vi "XML Parser Scheds.vi"(8 "error in (no error)":errorcluster, 11 "Schedule Filename":string) -> (0 "error out":errorcluster, 3 "output array":string[][](array[string]))   [LabVIEW 2023]
uses:
  <vilib>/xml/Close Reference(Node).vi
  <vilib>/xml/NI_XML.lvlib
  <resource>/objmgr/DOMUserDefRef.rc
panel:
  out "XML":string
  out "Parse Errors":string
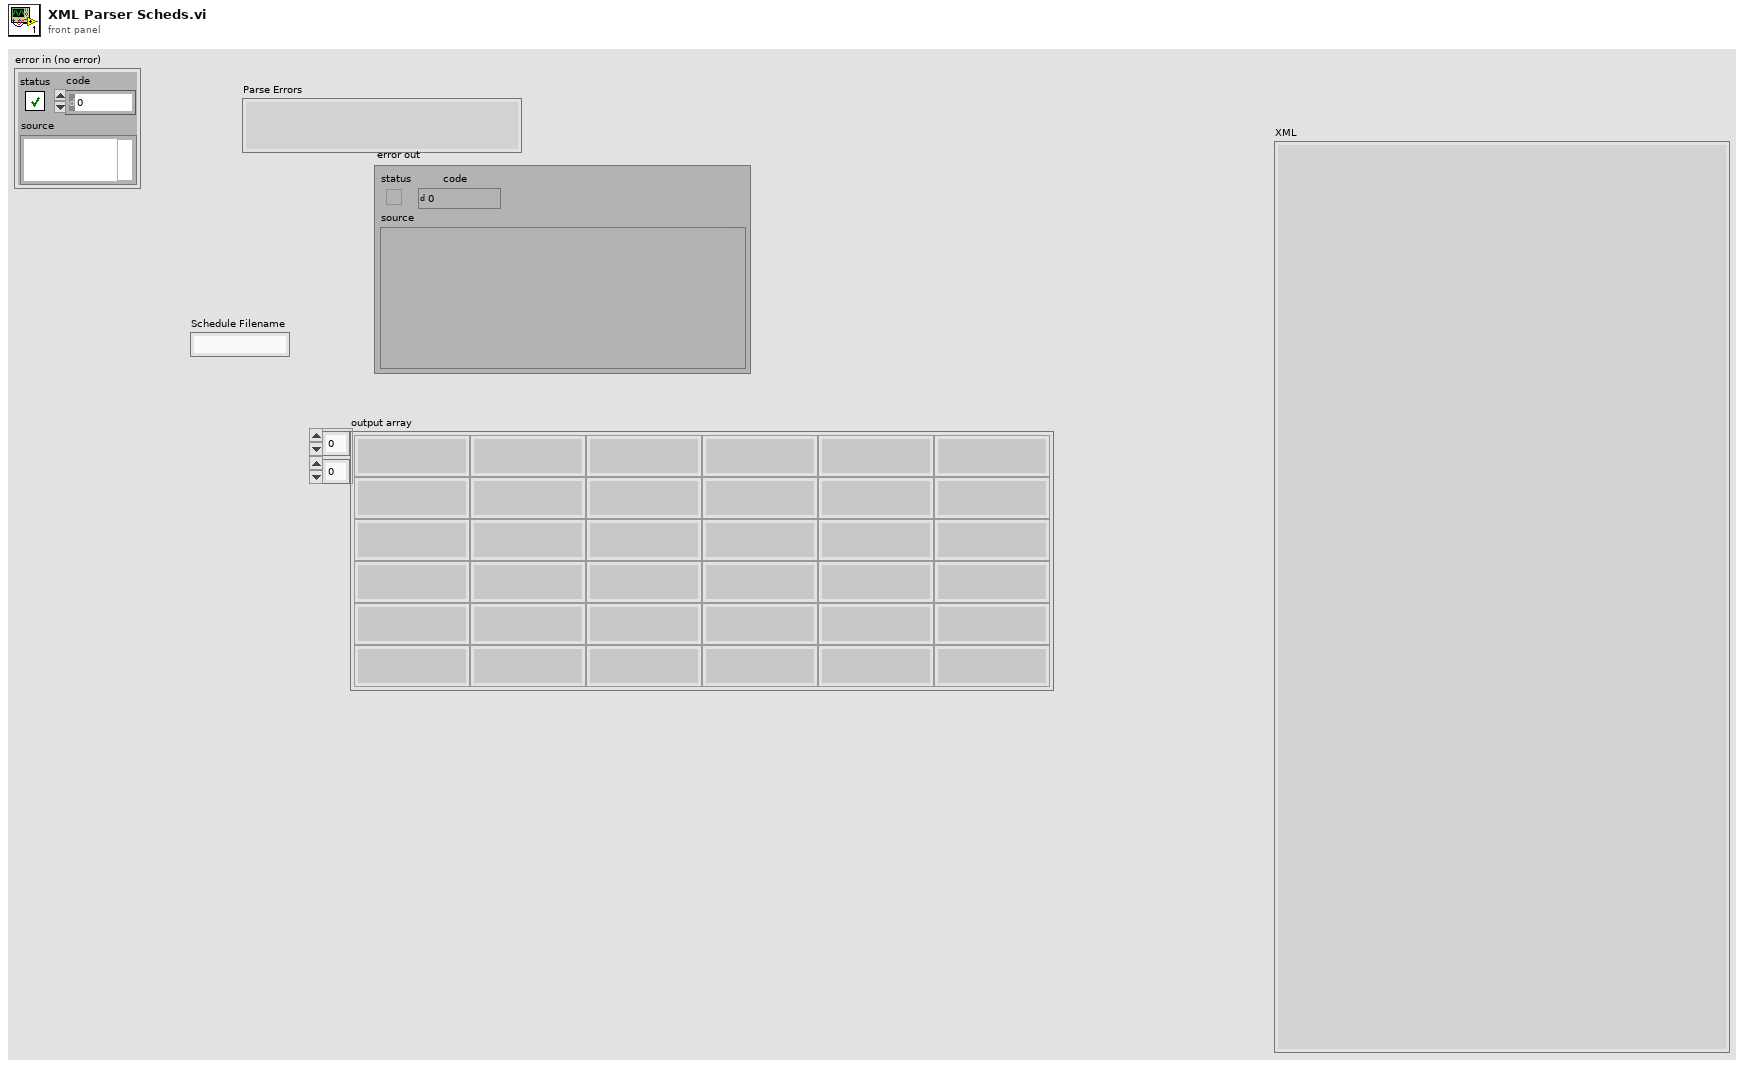
[diagram p1: front panel]
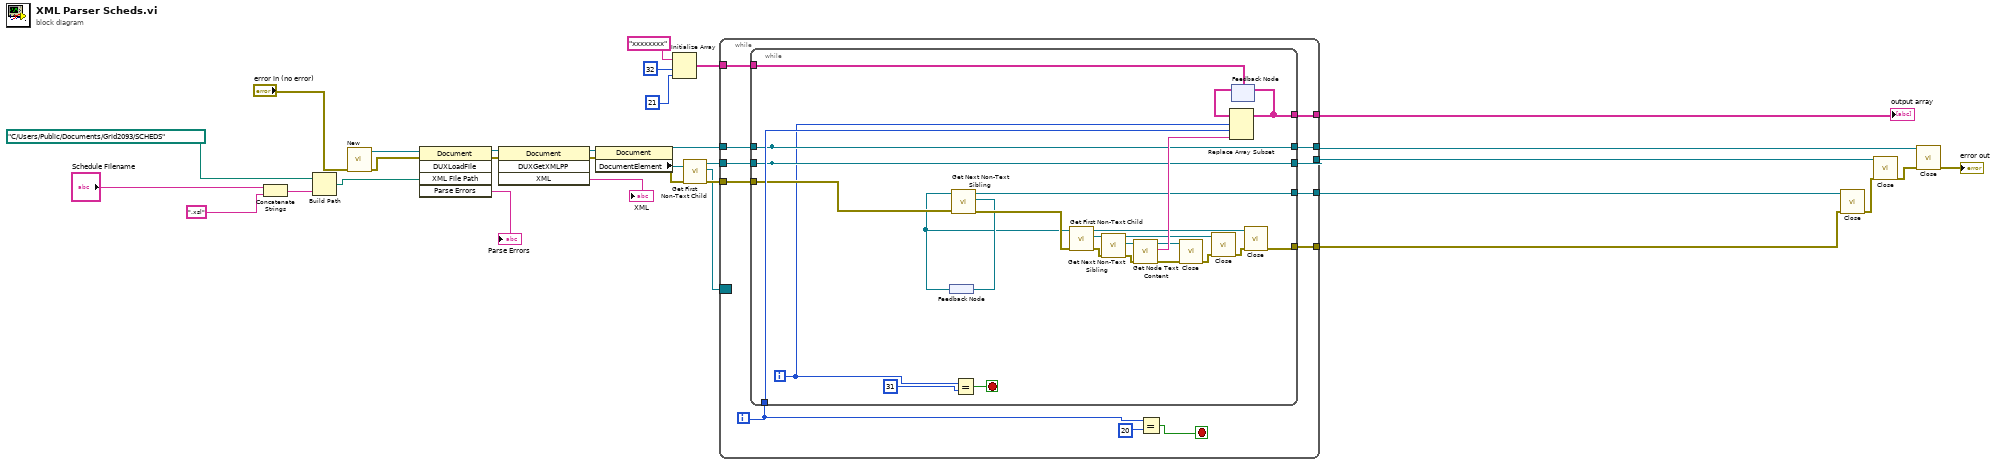
[diagram p0: block diagram]
diagram:
  n1 = Concatenate Strings("Schedule Filename", ".xsl" ("string")) -> (w23:string)
  n2 = Build Path(base path=path "C:/Users/Public/Documents/Grid2093/SCHEDS", name or relative path=w23) -> (appended path=w22:path)
  n3 = call <vilib>:"New.vi"("error in (no error)"="error in (no error)") -> ("error out"=w31:errorcluster, "DOM document out"=w32:refnum<k20>)  [unwired: 7 in]
  n4 = invoke class="Document" method="DUXLoadFile"(reference=w32, error in=w31, "XML File Path"=w22) -> (reference out=w30:refnum<k20>, error out=w29:errorcluster, "Parse Errors"=→"Parse Errors":string)  [unwired: 2 in, 2 out]
  n5 = invoke class="Document" method="DUXGetXMLPP"(reference=w30, error in=w29) -> (reference out=w28:refnum<k20>, error out=w27:errorcluster, "XML"=→"XML":string)  [unwired: 2 in, 1 out]
  n6 = property class="Document"(reference=w28, error in=w27) -> (reference out=w16:refnum<k20>, error out=w17:errorcluster, "DocumentElement"=w18:refnum<k20>)
  n7 = Initialize Array("xxxxxxxx", 32 ("dimension size"), 21 ("dimension size")) -> (w12:string[][])
  n8 = call <vilib>:"Get First Non-Text Child.vi"("error in (no error)"=w17, "node in"=w18) -> ("error out"=w10:errorcluster, "child node"=w1:refnum<k20>, "node out"=w11:refnum<k20>)  [unwired: 6 in, 1 out]
  n9 = while {
    tunnel: w16 -> [w44]
    tunnel: w10 -> [w43]
    tunnel: w11 -> [w42]
    tunnel: w12 -> [w41]
    tunnel: [w40] -> w9
    tunnel: [w39] -> w8
    tunnel: [w38] -> w4
    tunnel: [w34] -> w3
    tunnel: [w33] -> w5
    border: w1 -> [_]
    i -> [w35]
    stop <- w37 stop-if-true
    n10 = while {
      tunnel: w44 -> [w68]
      tunnel: w43 -> [w66]
      tunnel: w42 -> [w67]
      tunnel: w41 -> [w65]
      tunnel: w35 -> [w69]
      tunnel: [w68] -> _
      tunnel: [w67] -> _
      tunnel: [w68] -> w40
      tunnel: [w67] -> w39
      tunnel: [w47] -> w38
      tunnel: [w49] -> w34
      tunnel: [w48] -> w33
      i -> [w52]
      stop <- w51 stop-if-true
      n11 = feedback #1() -> (w45:refnum<k20>)
      n12 = call <vilib>:"Get Next Non-Text Sibling.vi"("error in (no error)"=w66, "node in"=w45) -> ("error out"=w54:errorcluster, "sibling node"=w46:refnum<k20>, "node out"=w48:refnum<k20>)  [unwired: 6 in, 1 out]
      n13 = feedback-in #1(w46) -> ()
      n14 = Equal?(x=w52, y=31) -> (x = y?=w51:bool)
      n15 = call <vilib>:"Get First Non-Text Child.vi"("error in (no error)"=w54, "node in"=w45) -> ("error out"=w61:errorcluster, "child node"=w62:refnum<k20>, "node out"=w56:refnum<k20>)  [unwired: 6 in, 1 out]
      n16 = call <vilib>:"Get Next Non-Text Sibling.vi"("error in (no error)"=w61, "node in"=w62) -> ("error out"=w59:errorcluster, "sibling node"=w60:refnum<k20>, "node out"=w58:refnum<k20>)  [unwired: 6 in, 1 out]
      n17 = call <vilib>:"Get Node Text Content.vi"("error in (no error)"=w59, "node in"=w60) -> ("error out"=w64:errorcluster, "node text"=w70:string, "node out"=w63:refnum<k20>)  [unwired: 7 in]
      n18 = call-poly <vilib>:"Close.vi"("error in (no error)"=w64, "node"=w63) -> ("error out"=w57:errorcluster)  [unwired: 7 in]
      n19 = call-poly <vilib>:"Close.vi"("error in (no error)"=w57, "node"=w58) -> ("error out"=w55:errorcluster)  [unwired: 7 in]
      n20 = feedback #2(w65) -> (w50:string[][])
      n21 = Replace Array Subset(array=w50, new element=w70, index (row)=w52, index (col)=w69) -> (w47:string[][])
      n22 = feedback-in #2(w47) -> ()
      n23 = call-poly <vilib>:"Close.vi"("error in (no error)"=w55, "node"=w56) -> ("error out"=w49:errorcluster)  [unwired: 7 in]
    }
    n24 = Equal?(x=w35, y=20 ("x")) -> (x = y?=w37:bool)
  }
  "output array" <- w4
  n25 = call-poly <vilib>:"Close.vi"("error in (no error)"=w3, "node"=w5) -> ("error out"=w6:errorcluster)  [unwired: 7 in]
  n26 = call-poly <vilib>:"Close.vi"("error in (no error)"=w6, "node"=w8) -> ("error out"=w7:errorcluster)  [unwired: 7 in]
  n27 = call-poly <vilib>:"Close.vi"("error in (no error)"=w7, "node"=w9) -> ("error out"=→"error out":errorcluster)  [unwired: 7 in]
